vi "Parsing Vision Result For Set.vi"(11 "VisionProject":u16) -> (2 "Dataout":string, 3 "DataoutName":string)   [LabVIEW 2019]
uses:
  8467066c-a009-426f-a9ca-a92f8a38ba5b.vi
  c9bb6bb5-397f-4184-9042-3819e11fa811.vi
  <vilib>/JDP Science/JSONtext/JSON text to Variant.vi
panel:
  out "Data out 2":string[][](array[string])
  out "Data out":string[][](array[string])
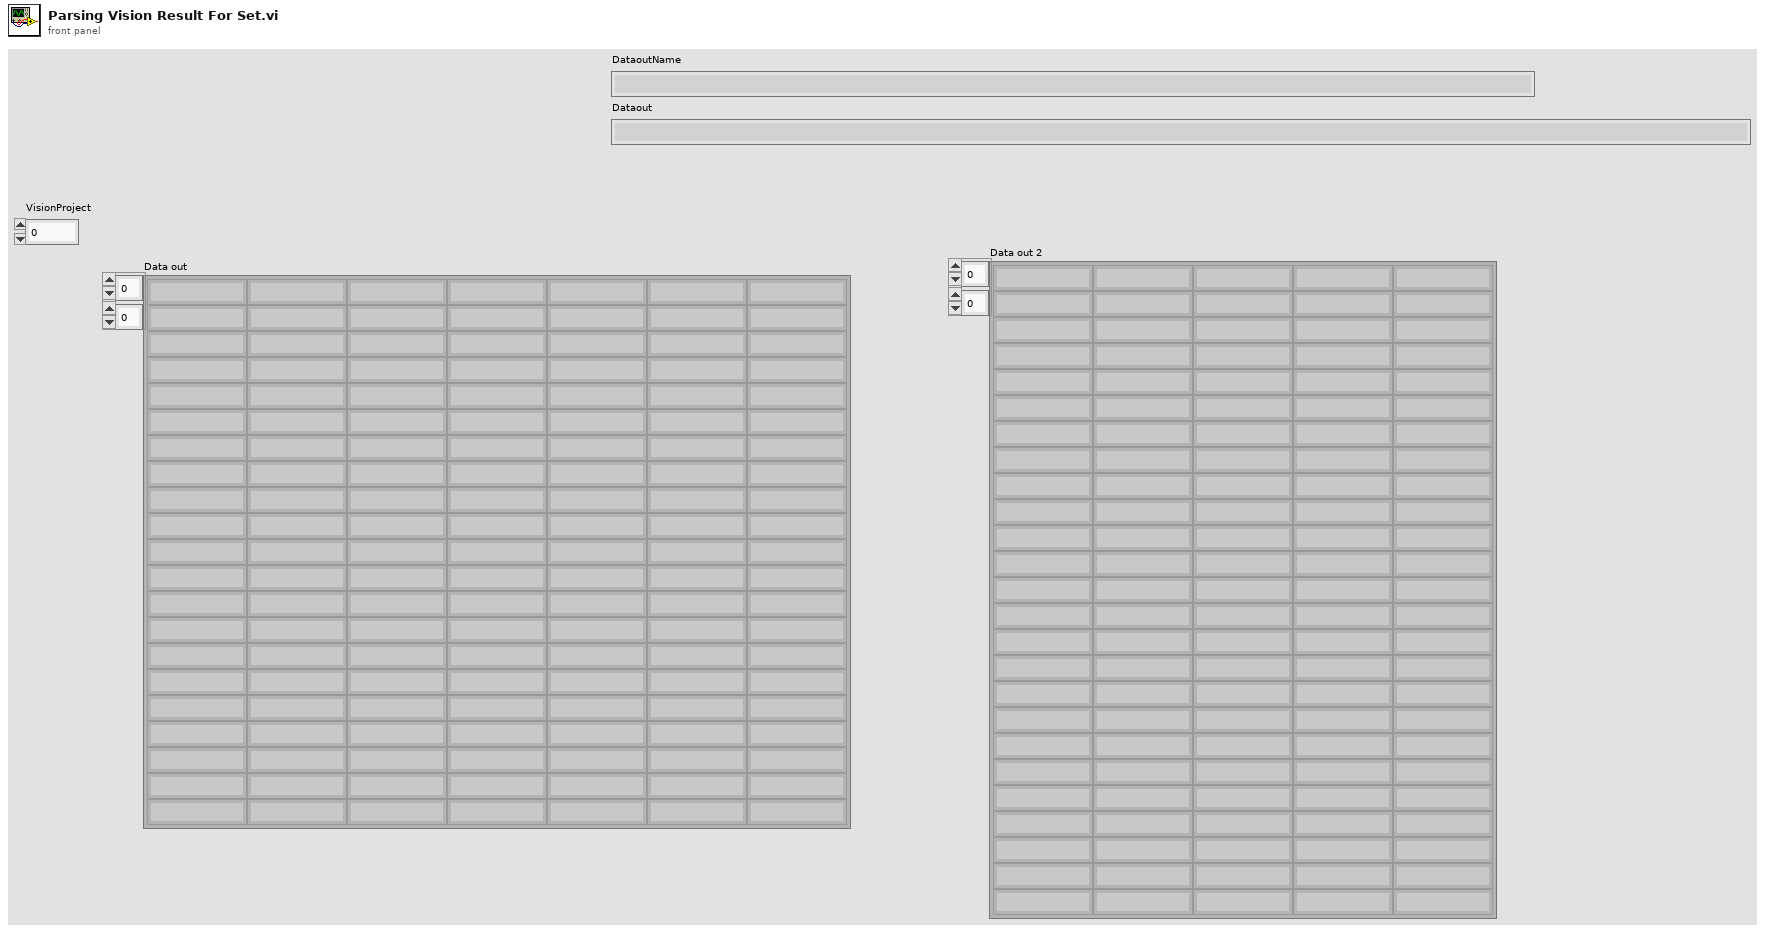
[diagram p1: front panel]
types:
  T1 = enum16{"initial", "write", "add", "delete", "Load", "Save", "Read", "ReadProjectName"}
  T2 = cluster{"ProjectName":string, "Parameter":string[][]}
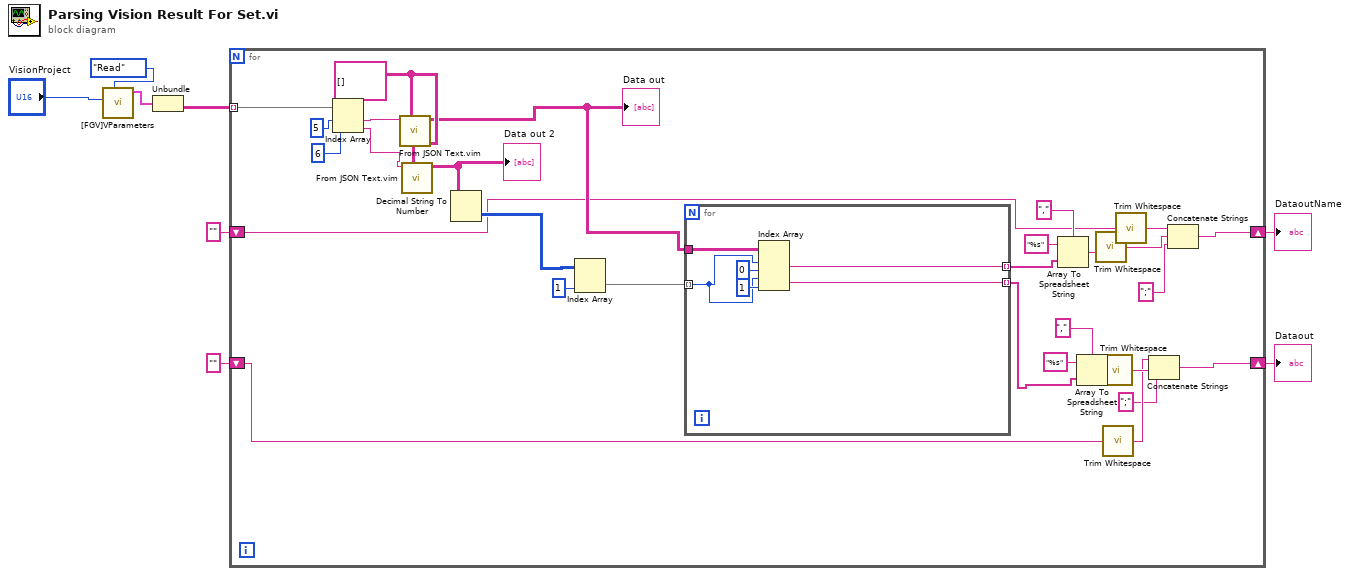
[diagram p0: block diagram]
diagram:
  n1 = call "[FGV]VParameters.vi"("Enum"=T1."Read", "ProjectIndex"="VisionProject") -> ("DataOut"=w7:T2)  [unwired: 6 in, 3 out]
  n2 = Unbundle(w7) -> ("Parameter"=w8:string[][])  [unwired: 1 out]
  n3 = for {
    tunnel: w8 -> [w37] mode=indexing
    shift-right: [w16] -> w2
    shift-left: "" -> [w20]
    shift-right: [w18] -> w1
    shift-left: "" -> [w17]
    w32 = string[][] []
    n4 = Index Array(array=w37, index #1=5 ("disabled index (col)"), index #2=6 ("disabled index (col)")) -> (element #1=w34:string, element #2=w33:string)
    n5 = call "From JSON Text.vim"("Data Type and Default Value"=w32, "JSON"=w34) -> ("Data out"=w27:string[][])  [unwired: 8 in, 1 out]
    "Data out" <- w27
    n6 = call "From JSON Text.vim"("Data Type and Default Value"=w32, "JSON"=w33) -> ("Data out"=w31:string[][])  [unwired: 8 in, 1 out]
    "Data out 2" <- w31
    n7 = Decimal String To Number(string=w31) -> (number=w29:i32[][])  [unwired: 2 in, 1 out]
    n8 = Index Array(array=w29, index (col)=1 ("disabled index (col)")) -> (element=w28:i32[])  [unwired: 1 in]
    n9 = for {
      tunnel: w28 -> [w40] mode=indexing
      tunnel: w27 -> [w43]
      tunnel: [w39] -> w26 mode=indexing
      tunnel: [w38] -> w21 mode=indexing
      n10 = Index Array(array=w43, index (row) #1=w40, index (col) #1=0 ("disabled index (col)"), index (row) #2=w40, index (col) #2=1 ("index (col)")) -> (element #1=w39:string, element #2=w38:string)
    }
    n11 = Array To Spreadsheet String(delimiter (Tab)=",", array=w26, 3:"%s" ("format string")) -> (spreadsheet string=w15:string)
    n12 = Array To Spreadsheet String(delimiter (Tab)=",", array=w21, 3:"%s" ("format string")) -> (spreadsheet string=w19:string)
    n13 = call <vilib>:"Trim Whitespace.vi"("string"=w15) -> ("trimmed string"=w13:string)  [unwired: 1 in]
    n14 = call <vilib>:"Trim Whitespace.vi"("string"=w19) -> ("trimmed string"=w12:string)  [unwired: 1 in]
    n15 = call <vilib>:"Trim Whitespace.vi"("string"=w17) -> ("trimmed string"=w11:string)  [unwired: 1 in]
    n16 = call <vilib>:"Trim Whitespace.vi"("string"=w20) -> ("trimmed string"=w14:string)  [unwired: 1 in]
    n17 = Concatenate Strings(w11, w12, ";" ("string")) -> (w18:string)
    n18 = Concatenate Strings(w14, w13, ";" ("string")) -> (w16:string)
  }
  "DataoutName" <- w2
  "Dataout" <- w1
